vi "Read CRD DVR.vi"(8 "error in (no error)":errorcluster, 11 "Calibration UI in":refnum<class "Calibration UI.lvclass">) -> (0 "error out":errorcluster, 2 "CRD DVR":refnum<data-value>, 3 "Calibration UI out":refnum<class "Calibration UI.lvclass">)   [LabVIEW 2015, in "Calibration UI.lvclass"]
uses:
  Calibration UI.lvclass
  CRDS/Data/cCRDS Data.lvclass
  Calibration UI.lvclass/Calibration UI.ctl
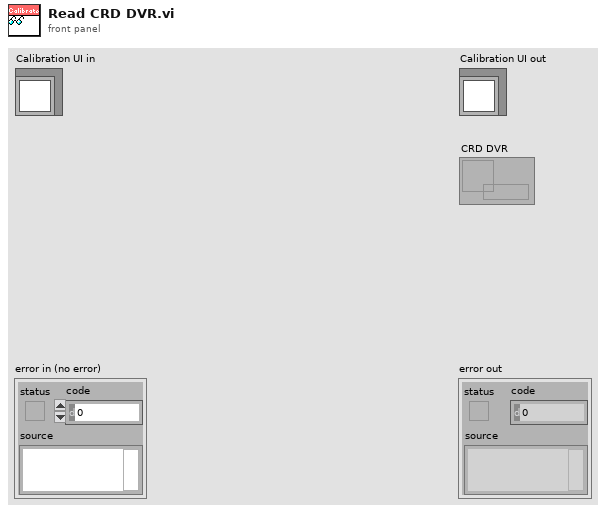
[diagram p1: front panel]
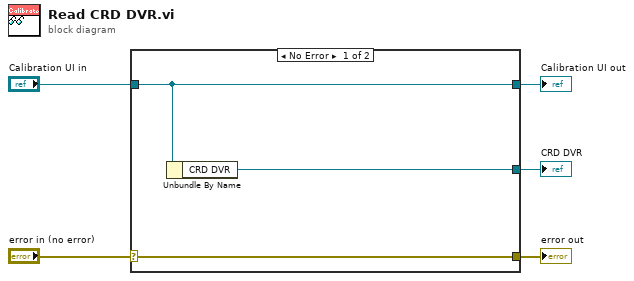
[diagram p0: block diagram]
diagram:
  n1 = case shown="No Error" "error in (no error)" {
    selector: "error in (no error)" -> [w8 w9]
    tunnel: [w8 w9] -> w4
    tunnel: [w7 w10] -> w2
    tunnel: "Calibration UI in" -> [w7 w10]
    tunnel: [w6 _] -> w1
    frame No Error {
      n2 = Unbundle By Name(w7) -> ("CRD DVR"=w6:refnum<data-value>)
    }
    frame Error {
    }
  }
  "error out" <- w4
  "Calibration UI out" <- w2
  "CRD DVR" <- w1
